vi "Write.vi"(8 "error in (no error)":errorcluster, 10 "Write Buffer (\"\")":string, 11 "VISA resource name":refnum<visa-resource-name>) -> (0 "error out":errorcluster, 3 "VISA resource name out":refnum<visa-resource-name>)   [LabVIEW 2013, in "RIGOL DP800 Series.lvlib"]
doc: "Writes the data from write buffer to the device or interface specified by VISA resource name."
uses:
  <instrlib>/RIGOL DP800 Series/RIGOL DP800 Series.lvlib
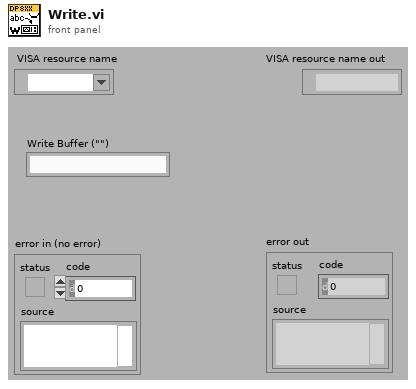
[diagram p1: front panel]
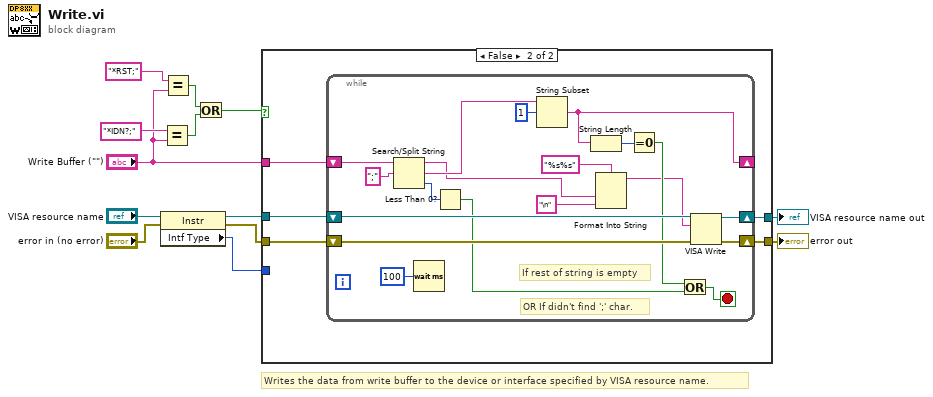
[diagram p0: block diagram]
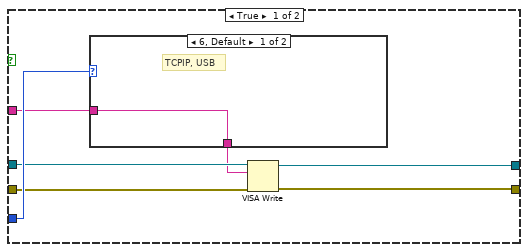
[diagram p2: hidden frame]
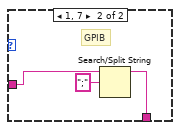
[diagram p3: hidden frame]
diagram:
  # "Writes the data from write buffer to the device or interface specified by VISA resource name."
  n1 = property class="Instr"(reference="VISA resource name", error in="error in (no error)") -> (reference out=w2:refnum<visa-resource-name>, error out=w3:errorcluster, "Intf Type"=w1:u16)
  n2 = Equal?(x="*IDN?;", y="Write Buffer (\"\")") -> (x = y?=w8:bool)
  n3 = Equal?(x="*RST;", y="Write Buffer (\"\")") -> (x = y?=w7:bool)
  n4 = Or(x=w7, y=w8) -> (x .or. y?=w6:bool)
  n5 = case shown="False" w6 {
    tunnel: w2 -> [w18 w29]
    tunnel: w3 -> [w17 w28]
    tunnel: [w15 w27] -> w13
    tunnel: [w16 w26] -> w12
    tunnel: "Write Buffer (\"\")" -> [w19 w25]
    tunnel: w1 -> [w20 _]
    frame True {
      n6 = case shown="6, Default" w20 {
        tunnel: [w21 w22] -> w14
        tunnel: w19 -> [w21 w24]
        frame 6, Default {
          # "TCPIP, USB"
        }
        frame 1, 7 {
          # "GPIB"
          n7 = Search/Split String(string=w24, search string/char (-)=";") -> (substring before match=w22:string)  [unwired: 1 in, 2 out]
        }
      }
      n8 = VISA Write(VISA resource name=w18, write buffer=w14, error in (no error)=w17) -> (VISA resource name out=w15:refnum<visa-resource-name>, error out=w16:errorcluster)  [unwired: 1 out]
    }
    frame False {
      n9 = while {
        shift-right: [w46] -> w27
        shift-left: w29 -> [w48]
        shift-right: [w45] -> w26
        shift-left: w28 -> [w47]
        shift-right: [w39] -> _
        shift-left: w25 -> [w43]
        stop <- w37 stop-if-true
        # "OR If didn't find ';' char."
        # "If rest of string is empty"
        n10 = Search/Split String(string=w43, search string/char (-)=";") -> (substring before match=w32:string, match + rest of string=w41:string, offset of match=w42:i32)  [unwired: 1 in]
        n11 = Wait (ms)(milliseconds to wait=u32 100) -> ()  [unwired: 1 out]
        n12 = Less Than 0?(x=w42) -> (x < 0?=w36:bool)
        n13 = String Subset(string=w41, offset (0)=1) -> (substring=w39:string)  [unwired: 1 in]
        n14 = String Length(string=w39) -> (length=w38:i32)
        n15 = Format Into String(format string="%s%s", w32, "\n" ("string")) -> (resulting string=w30:string)  [unwired: 2 in, 1 out]
        n16 = Equal To 0?(x=w38) -> (x = 0?=w35:bool)
        n17 = Or(x=w35, y=w36) -> (x .or. y?=w37:bool)
        n18 = VISA Write(VISA resource name=w48, write buffer=w30, error in (no error)=w47) -> (VISA resource name out=w46:refnum<visa-resource-name>, error out=w45:errorcluster)  [unwired: 1 out]
      }
    }
  }
  "VISA resource name out" <- w13
  "error out" <- w12
